vi "Write to Excel multiple data.vi"() -> ()   [LabVIEW 2022 SP3]
panel:
  in  "Cluster":T1
  out "error out":errorcluster
  in  "file path (use dialog)":path
  out "Waveform Graph":dbl[](graph)
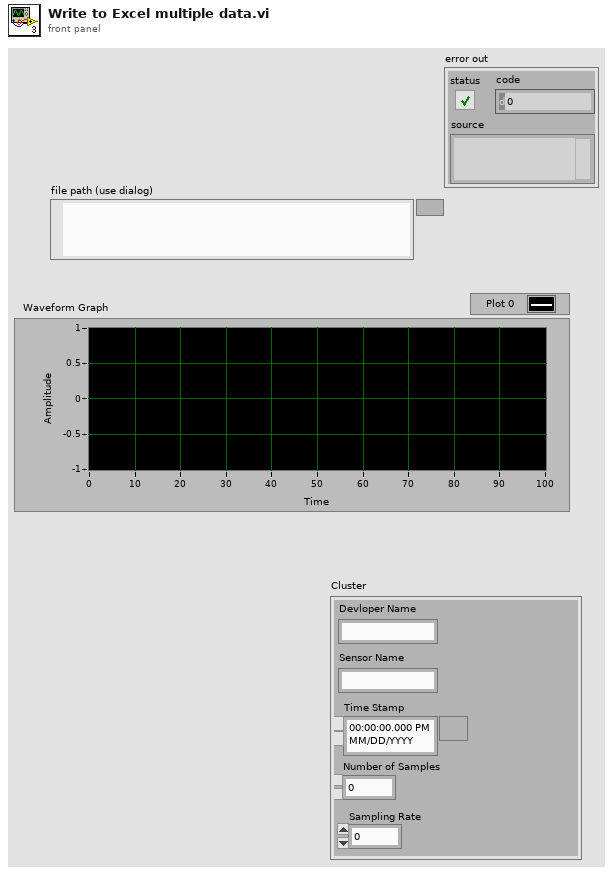
[diagram p1: front panel]
types:
  T1 = cluster{"Devloper Name ":string, "Sensor Name":string, "Time Stamp":timestamp, "Number of Samples":dbl, "Sampling Rate":dbl}
  T2 = enum16{"open", "replace", "create", "open or create", "replace or create", "replace or create with confirmation"}
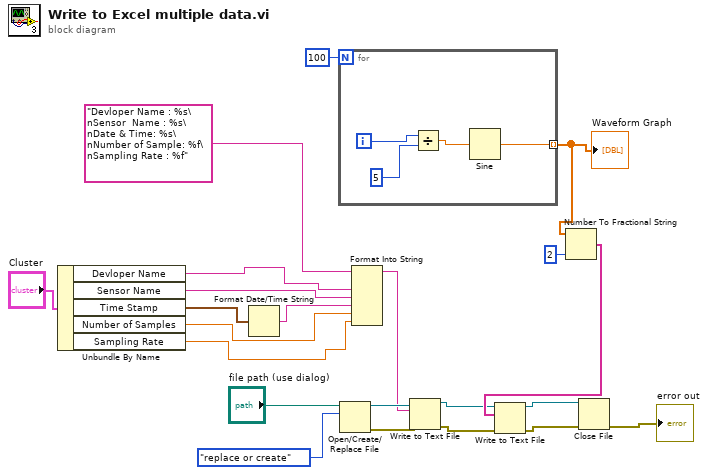
[diagram p0: block diagram]
diagram:
  n1 = Unbundle By Name("Cluster") -> ("Devloper Name"=w5:string, "Sensor Name"=w4:string, "Time Stamp"=w3:timestamp, "Number of Samples"=w2:dbl, "Sampling Rate"=w1:dbl)
  n2 = Format Date/Time String(seconds (now)=w3) -> (date/time string=w7:string)  [unwired: 2 in]
  n3 = for {
    N: 100 -> [_]
    tunnel: [w23] -> w15 mode=indexing
    i -> [w26]
    n4 = Divide(x=w26, y=5) -> (x/y=w24:dbl)
    n5 = Sine(x=w24) -> (sin(x)=w23:dbl)
  }
  "Waveform Graph" <- w15
  n6 = Open/Create/Replace File(file path (use dialog)="file path (use dialog)", operation (0:open)=T2."replace or create") -> (refnum out=w13:refnum<file>, error out=w12:errorcluster)  [unwired: 4 in, 1 out]
  n7 = Format Into String(format string="Devloper Name : %s\nSensor  Name : %s\nDate & Time: %s\nNumber of Sample: %f\nSampling Rate : %f", w5, w4, w7, w2, w1) -> (resulting string=w9:string)  [unwired: 2 in, 1 out]
  n8 = Write to Text File(file (use dialog)=w13, text=w9, error in=w12) -> (refnum out=w10:refnum<file>, error out=w11:errorcluster)  [unwired: 1 in, 1 out]
  n9 = Number To Fractional String(number=w15, precision (6)=i16 2) -> (F-format string=w14:string[])  [unwired: 2 in]
  n10 = Write to Text File(file (use dialog)=w10, text=w14, error in=w11) -> (refnum out=w19:refnum<file>, error out=w18:errorcluster)  [unwired: 1 in, 1 out]
  n11 = Close File(refnum=w19, error in=w18) -> (error out=→"error out":errorcluster)  [unwired: 1 out]
